vi "作业2按钮事件结构.vi"() -> ()   [LabVIEW 2017]
panel:
  out "数值":dbl
  in  "停止":bool
  in  "按钮 3":bool
  in  "按钮 2":bool
  in  "按钮1":bool
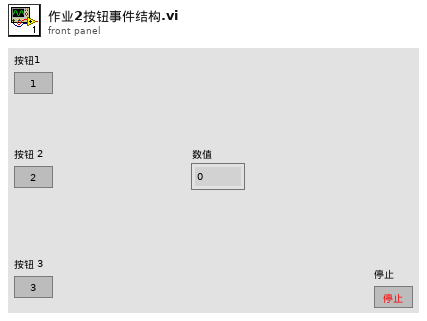
[diagram p1: front panel]
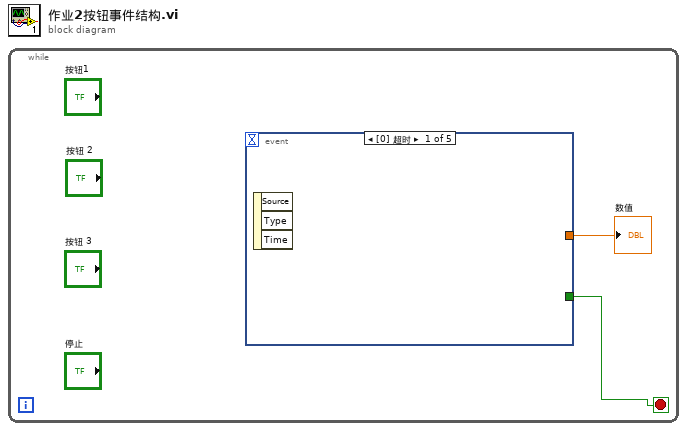
[diagram p0: block diagram]
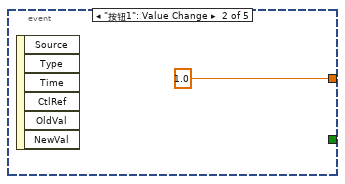
[diagram p2: hidden frame]
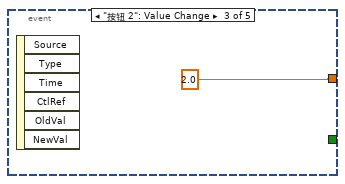
[diagram p3: hidden frame]
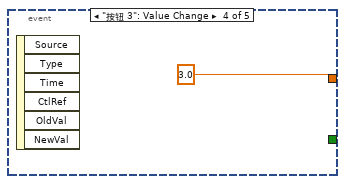
[diagram p4: hidden frame]
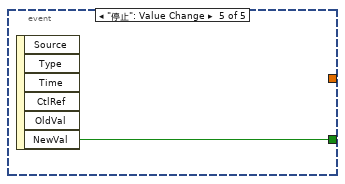
[diagram p5: hidden frame]
diagram:
  n1 = while {
    stop <- w1 stop-if-true
    n2 = event "事件结构" shown="[0] 超时" {
      selector: _ -> [_ _ _ _ _]
      dyn-events: _ -> [_ _ _ _ _]
      timeout: _ -> [_ _ _ _ _]
      tunnel: [_ 1.0 2.0 3.0 _] -> w2
      tunnel: [_ _ _ _ w6] -> w1
      event Timeout {
        n3 = event-data() -> ()  [unwired: 1 in, 3 out]
      }
      event "按钮1": Value Change {
        n4 = event-data() -> ()  [unwired: 1 in, 6 out]
      }
      event "按钮 2": Value Change {
        n5 = event-data() -> ()  [unwired: 1 in, 6 out]
      }
      event "按钮 3": Value Change {
        n6 = event-data() -> ()  [unwired: 1 in, 6 out]
      }
      event "停止": Value Change {
        n7 = event-data() -> ("NewVal"=w6:bool)  [unwired: 1 in, 5 out]
      }
    }
    "数值" <- w2
  }
